vi "gvboolesch.vi"() -> ()   [LabVIEW 2010]
panel:
  in  "Rampe 2 los Mach 2":bool
  in  "Kühlen los Mach 2":bool
  in  "Rampe los Mach 2":bool
  in  "Kühlen los Trap 2":bool
  in  "Rampe los Trap 2":bool
  in  "Rampe 2 los Mach":bool
  in  "Kühlen los Trap":bool
  in  "Rampe los Trap":bool
  in  "Kühlen los Mach":bool
  in  "Rampe los Mach":bool
  in  "global stop":bool
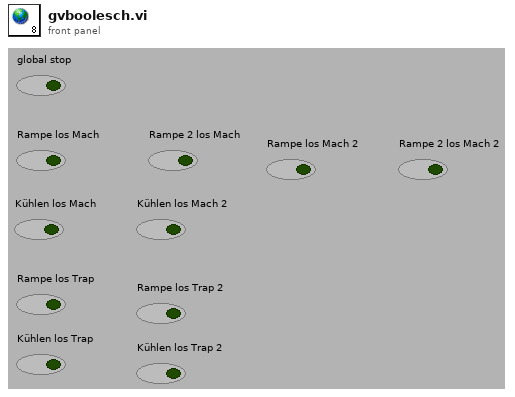
[diagram p1: front panel]
diagram:
